vi "Write IVI Resource.vi"(8 "error in (no error)":errorcluster, 10 "IVI Resource":refnum<k15>, 11 "PXIe5413 in":refnum<class "PXIe5413.lvclass">) -> (0 "error out":errorcluster, 3 "PXIe5413 out":refnum<class "PXIe5413.lvclass">)   [LabVIEW 2018, in "PXIe5413.lvlib" / "PXIe5413.lvclass"]
uses:
  PXIe5413.lvclass
  PXIe5413.lvclass/PXIe5413.ctl
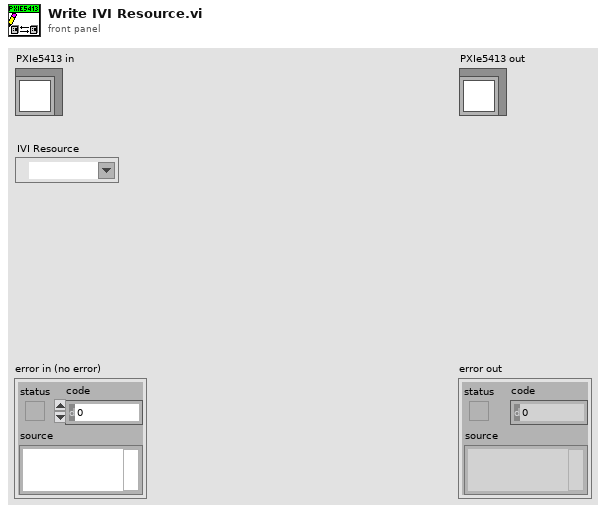
[diagram p1: front panel]
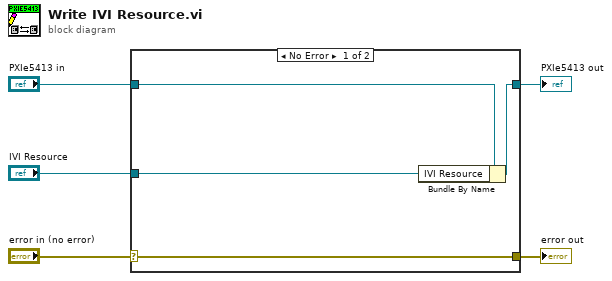
[diagram p0: block diagram]
diagram:
  n1 = case shown="No Error" "error in (no error)" {
    selector: "error in (no error)" -> [w9 w10]
    tunnel: [w9 w10] -> w4
    tunnel: [w7 w11] -> w2
    tunnel: "PXIe5413 in" -> [w8 w11]
    tunnel: "IVI Resource" -> [w6 _]
    frame No Error {
      n2 = Bundle By Name(cluster=w8, "IVI Resource"=w6) -> (w7:refnum<class "PXIe5413.lvclass">)
    }
    frame Error {
    }
  }
  "error out" <- w4
  "PXIe5413 out" <- w2
